vi "GetTimeCount1_ReentrantClone.vi"(8 "error IN":errorcluster) -> (0 "error OUT":errorcluster, 2 "[OUT] Timer Count":u32)   [LabVIEW 2020]
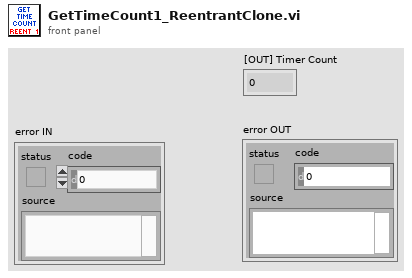
[diagram p1: front panel]
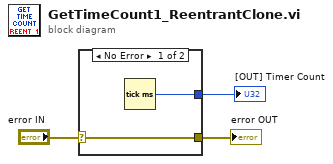
[diagram p0: block diagram]
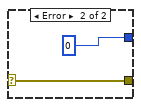
[diagram p2: hidden frame]
diagram:
  n1 = case shown="No Error" "error IN" {
    selector: "error IN" -> [w5 w7]
    tunnel: [w5 w7] -> w2
    tunnel: [w4 u32 0 ("millisecond timer value")] -> w1
    frame No Error {
      n2 = Tick Count (ms)() -> (millisecond timer value=w4:u32)
    }
    frame Error {
    }
  }
  "error OUT" <- w2
  "[OUT] Timer Count" <- w1
